vi "Create Monitor Log.vi"(8 "error in":errorcluster, 11 "Monitor Log Directory (/home/lvuser/)":string="/home/lvuser/") -> (0 "error out":errorcluster, 3 "refnum out":refnum<file>)   [LabVIEW 2020, in "AIM ARINC 664 Engine.lvlib" / "Implementation.lvlib" / "Monitor Execution Unit.lvclass"]
uses:
  Monitor Execution Unit.lvclass
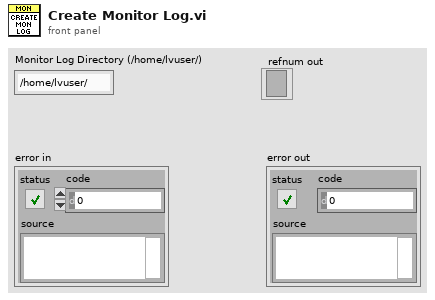
[diagram p1: front panel]
types:
  T1 = enum16{"open", "replace", "create", "open or create", "replace or create", "replace or create with confirmation"}
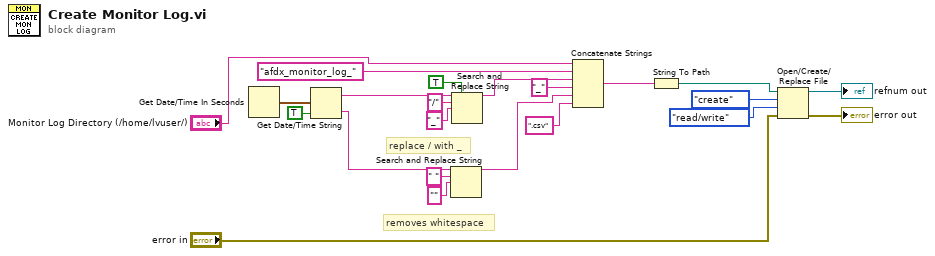
[diagram p0: block diagram]
diagram:
  # "removes whitespace"
  # "replace / with _"
  n1 = Get Date/Time In Seconds() -> (seconds since 1Jan1904=w17:timestamp)
  n2 = Get Date/Time String(seconds (now)=w17, want seconds? (F)=TRUE) -> (date string=w16:string, time string=w9:string)  [unwired: 1 in]
  n3 = Search and Replace String(input string=w9, search string=" ", replace string="" ("replace string (\"\")")) -> (result string=w8:string)  [unwired: 5 in, 3 out]
  n4 = Search and Replace String(replace all?=TRUE ("replace all? (F)"), input string=w16, search string="/", replace string="_" ("replace string (\"\")")) -> (result string=w15:string)  [unwired: 4 in, 3 out]
  n5 = Concatenate Strings("Monitor Log Directory (/home/lvuser/)", "afdx_monitor_log_" ("string"), w15, "_" ("string"), w8, ".csv" ("string")) -> (w18:string)
  n6 = String To Path(string=w18) -> (path=w20:path)
  n7 = Open/Create/Replace File(file path (use dialog)=w20, error in="error in", operation (0:open)=T1."create", access (0:read/write)=enum16{"read/write", "read-only", "write-only"}."read/write") -> (refnum out=→"refnum out":refnum<file>, error out=→"error out":errorcluster)  [unwired: 2 in, 1 out]
